vi "Save_UV-vis.vi"(8 "error in":errorcluster, 9 "measurement":ext[][](array[numeric]), 10 "step":ext, 11 "start":ext) -> (0 "error out":errorcluster)   [LabVIEW 2010]
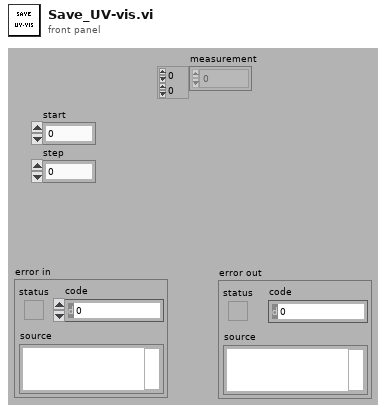
[diagram p1: front panel]
types:
  T1 = enum16{"open", "replace", "create", "open or create", "replace or create", "replace or create with confirmation"}
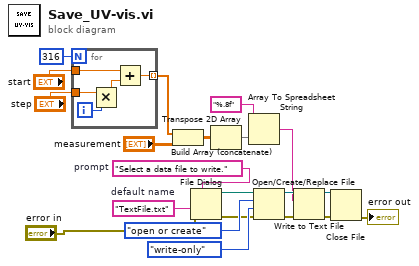
[diagram p0: block diagram]
diagram:
  w15 = "TextFile.txt"  # default name
  w16 = "Select a data file to write."  # prompt
  n1 = for {
    N: 316 -> [_]
    tunnel: "start" -> [w26]
    tunnel: "step" -> [w24]
    tunnel: [w22] -> w6 mode=indexing
    i -> [w25]
    n2 = Multiply(x=w24, y=w25) -> (x*y=w23:ext)
    n3 = Add(x=w26, y=w23) -> (x+y=w22:ext)
  }
  n4 = Build Array (concatenate)(w6, "measurement") -> (w9:ext[][])
  n5 = File Dialog(7:w16, 8:"error in", 9:w15) -> (0:w17:errorcluster, 3:w14:path)  [unwired: 6 out]
  n6 = Transpose 2D Array(2D array=w9) -> (transposed array=w11:ext[][])
  n7 = Array To Spreadsheet String(array=w11, 3:"%.8f") -> (spreadsheet string=w4:string)  [unwired: 1 out]
  n8 = Open/Create/Replace File(file path (use dialog)=w14, error in=w17, operation (0:open)=T1."open or create", access (0:read/write)=enum16{"read/write", "read-only", "write-only"}."write-only") -> (refnum out=w18:refnum<file>, error out=w19:errorcluster)  [unwired: 3 out]
  n9 = Write to Text File(file (use dialog)=w18, text=w4, error in=w19) -> (refnum out=w12:refnum<file>, error out=w13:errorcluster)  [unwired: 1 in, 1 out]
  n10 = Close File(refnum=w12, error in=w13) -> (error out=→"error out":errorcluster)  [unwired: 1 out]
